vi "計時器.vi"(4 "時間設定":dbl format="%#.6f", 6 "動作":bool) -> (0 "時間到":bool, 2 "計數時間":dbl format="%.2f", 3 "開始時間":dbl format="%.2f")   [LabVIEW 2015]
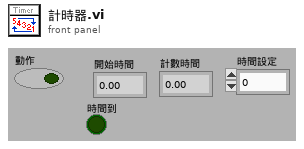
[diagram p1: front panel]
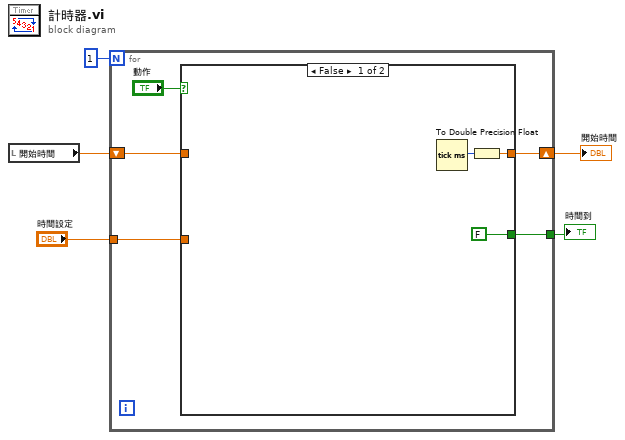
[diagram p0: block diagram]
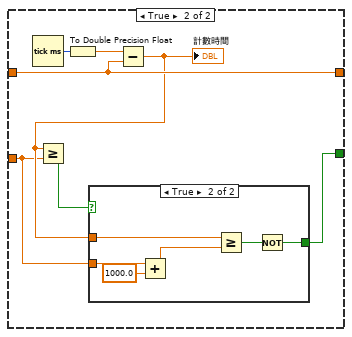
[diagram p2: hidden frame]
diagram:
  n1 = local read "開始時間"() -> (w3:dbl)
  n2 = for {
    N: 1 -> [_]
    shift-right: [w9] -> w4
    shift-left: w3 -> [w10]
    tunnel: "時間設定" -> [w7]
    tunnel: [w6] -> w1
    n3 = case shown="False" "動作" {
      tunnel: w10 -> [_ w20]
      tunnel: [w13 w20] -> w9
      tunnel: w7 -> [_ w14]
      tunnel: [FALSE w17] -> w6
      frame False {
        n4 = Tick Count (ms)() -> (millisecond timer value=w11:u32)
        n5 = To Double Precision Float(number=w11) -> (double precision float=w13:dbl)
      }
      frame True {
        n6 = Tick Count (ms)() -> (millisecond timer value=w19:u32)
        n7 = To Double Precision Float(number=w19) -> (double precision float=w16:dbl)
        n8 = Subtract(x=w16, y=w20) -> (x-y=w15:dbl)
        "計數時間" <- w15
        n9 = Greater Or Equal?(x=w15, y=w14) -> (x >= y?=w18:bool)
        n10 = case shown="True" w18 {
          selector: w18 -> [w21 _]
          tunnel: [w21 w22] -> w17
          tunnel: w14 -> [_ w27]
          tunnel: w15 -> [_ w25]
          frame False {
          }
          frame True {
            n11 = Add(x=w27, y=1000.0) -> (x+y=w24:dbl)
            n12 = Greater Or Equal?(x=w25, y=w24) -> (x >= y?=w23:bool)
            n13 = Not(x=w23) -> (.not. x?=w22:bool)
          }
        }
      }
    }
  }
  "開始時間" <- w4
  "時間到" <- w1
